vi "BezierGeneratorRev2Trans.vi"(1 "RobotY":dbl, 2 "RobotX":dbl, 3 "DeltaYaw":dbl, 4 "RobotOrientation":dbl=70.0, 5 "DeltaY":dbl=60.0, 6 "DeltaX":dbl=60.0) -> (0 "RobotNeededPathData":T1={"Path"=[], "MaxVel"=80.0, "MaxAccel"=100.0, "Backwards?"=FALSE, "PointSpacing"=6.0, "LookaheadDist"=13.0, "Speed/Curve"=1.8, "SlowDistanceAtEnd"=0.0, "SlowSpeed"=0.0, "MaxDeAccel"=80.0} {"SlowSpeed" format="%#_13g"; "SlowDistanceAtEnd" format="%#_13g"; "Speed/Curve" format="%#_13g"})   [LabVIEW 2018]
uses:
  Dawgma Programming Library/Controls/PurePursuit/RobotNeededPathData.ctl
panel:
  in  "SlowSpeed":dbl
  in  "SlowDistanceAtEnd":dbl
  in  "Speed/Curve":dbl=1.8
  in  "LookaheadDist":dbl=13.0
  in  "PointSpacing":dbl=6.0
  in  "MaxDeaccel":dbl=80.0
  in  "MaxAccel":dbl=100.0
  in  "MaxVel":dbl=80.0
  out "Curve":cluster{"X":dbl, "Y":dbl}[](graph)
  out "waypoints":cluster{dbl[], dbl[]}(graph)
  in  "TrajPointoffset":dbl=12.0
  in  "TargetOffset":dbl=12.0
  in  "Path":cluster{"x":dbl, "y":dbl}[](array[cluster])=[{"x"=0.0, "y"=0.0}, {"x"=0.0, "y"=0.0}, {"x"=0.0, "y"=0.0}, {"x"=0.0, "y"=0.0}]
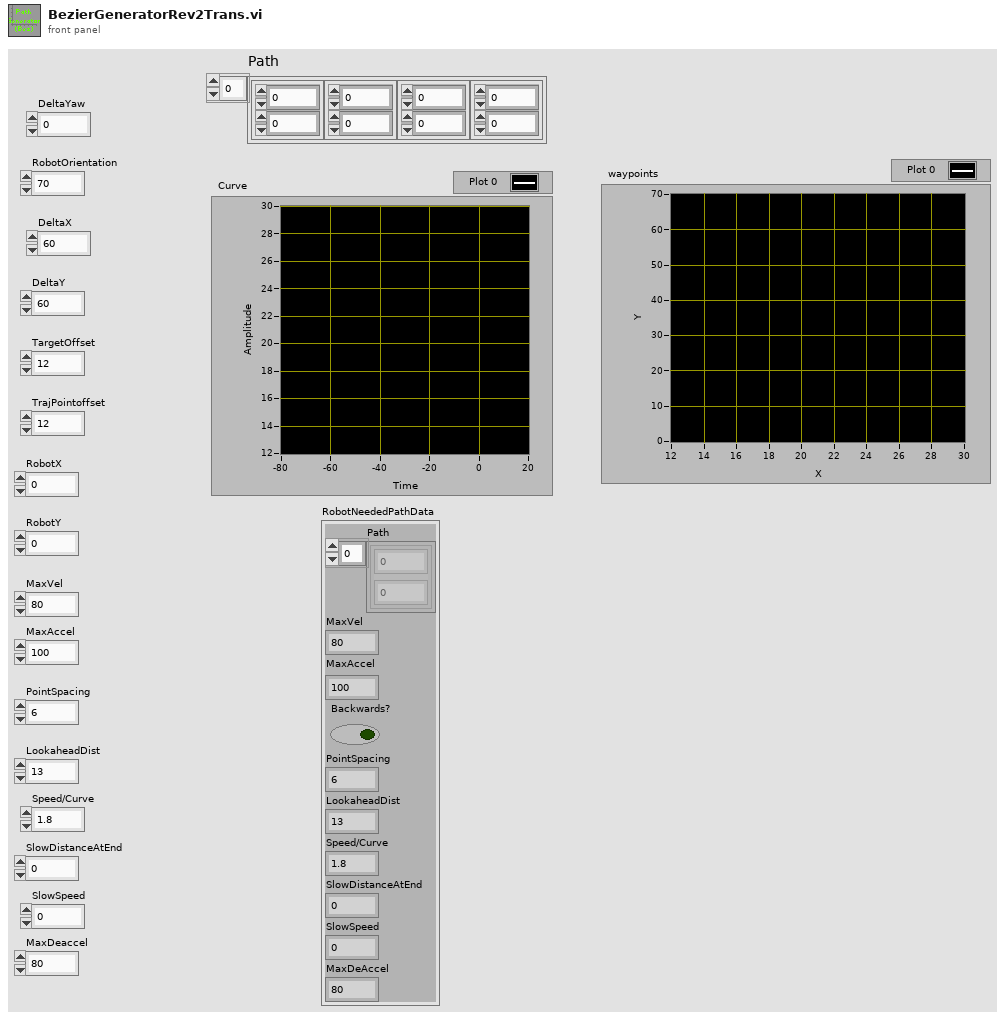
[diagram p1: front panel]
types:
  T1 = typedef "RobotNeededPathData.ctl" = cluster{"Path":cluster{dbl, dbl}[], "MaxVel":dbl, "MaxAccel":dbl, "Backwards?":bool, "PointSpacing":dbl, "LookaheadDist":dbl, "Speed/Curve":dbl, "SlowDistanceAtEnd":dbl, "SlowSpeed":dbl, "MaxDeAccel":dbl}
  T2 = cluster{"DeltaX":dbl, "DeltaY":dbl, "RobotOrientation":dbl, "TrajPointoffset":dbl, "TargetOffset":dbl, "DeltaYaw":dbl, "RobotX":dbl, "RobotY":dbl}
  T3 = cluster{cluster{"xP":dbl, "yP":dbl}[], "MaxVel":dbl, "MaxAccel":dbl, bool, "PointSpacing":dbl, "LookaheadDist":dbl, "Speed/Curve":dbl, "SlowDistanceAtEnd":dbl, "SlowSpeed":dbl, "MaxDeaccel":dbl}
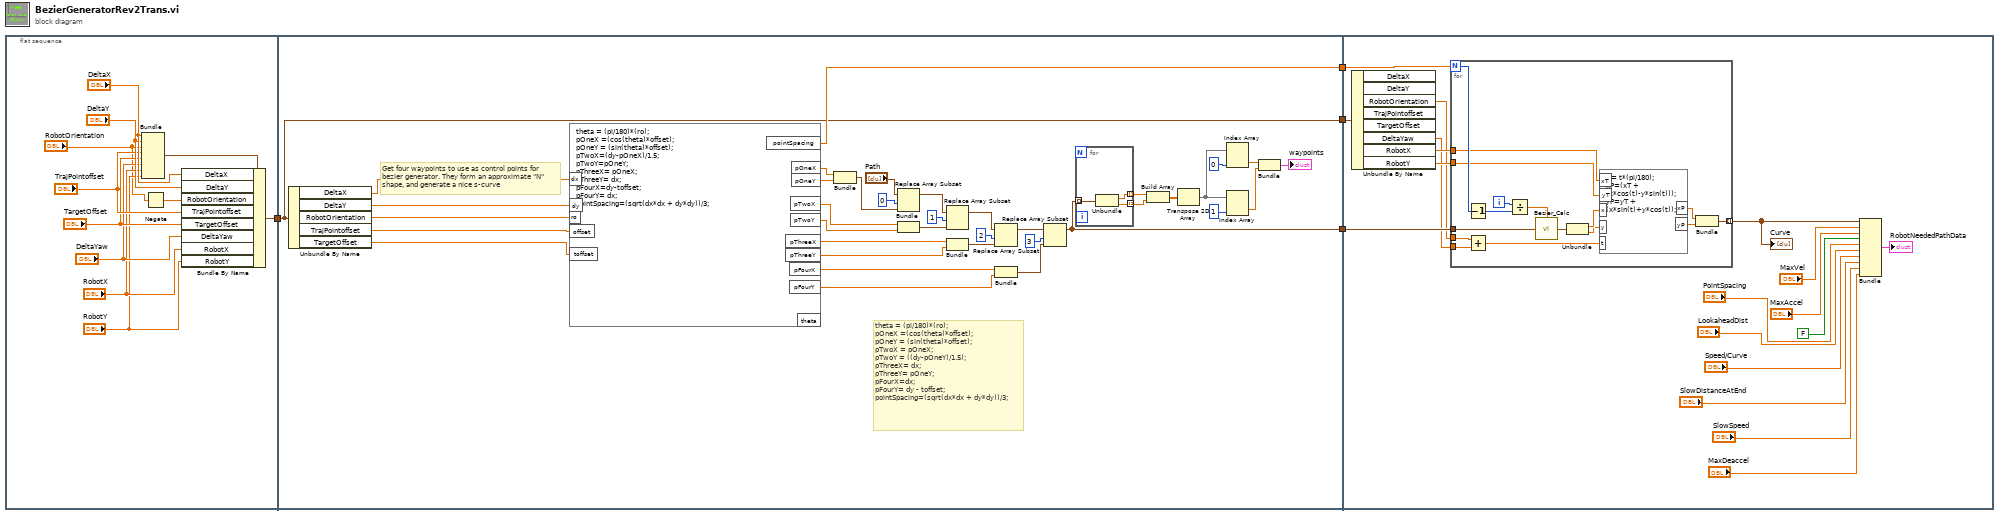
[diagram p0: block diagram]
diagram:
  n1 = flat-sequence {
    tunnel: [w14] -> w2
    tunnel: [w34] -> w4
    tunnel: [w23] -> w3
    tunnel: w2 -> [w16]
    tunnel: [w16] -> w1
    tunnel: w4 -> [w73]
    tunnel: w3 -> [w72]
    tunnel: w1 -> [w61]
    frame #0 {
      n2 = Bundle("DeltaX"="DeltaX", "DeltaY"="DeltaY", "RobotOrientation"="RobotOrientation", "TrajPointoffset"="TrajPointoffset", "TargetOffset"="TargetOffset", "DeltaYaw"="DeltaYaw", "RobotX"="RobotX", "RobotY"="RobotY") -> (w15:T2)  [unwired: 1 in]
      n3 = Negate(x="RobotOrientation") -> (-x=w5:dbl)
      n4 = Bundle By Name(cluster=w15, "DeltaX"="DeltaX", "DeltaY"="DeltaY", "RobotOrientation"=w5, "TrajPointoffset"="TrajPointoffset", "TargetOffset"="TargetOffset", "DeltaYaw"="DeltaYaw", "RobotX"="RobotX", "RobotY"="RobotY") -> (w14:T2)
    }
    frame #1 {
      # "theta = (pi/180)*(ro);\npOneX =(cos(theta)*offset);\npOneY = (sin(theta)*offset);\npTwoX = pOneX;\npTwoY = ((dy-pOneY)/1.5);\npThreeX= dx;\npThreeY= pOneY;\npFourX=dx;\npFourY= dy - toffset;\npointSpacing=(sqrt(dx*dx + dy*dy))/3;"
      # "Get four waypoints to use as control points for bezier generator. They form an approximate \"N\" shape, and generate a nice s-curve"
      n5 = Unbundle By Name(w16) -> ("DeltaX"=w28:dbl, "DeltaY"=w27:dbl, "RobotOrientation"=w24:dbl, "TrajPointoffset"=w25:dbl, "TargetOffset"=w26:dbl)
      n6 = formula code="theta = (pi/180)*(ro);\npOneX =(cos(theta)*offset);\npOneY = (sin(theta)*offset);\npTwoX=(dy-pOneX)/1.5;\npTwoY=pOneY;\npThreeX= pOneX;\npThreeY= dx;\npFourX=dy-toffset;\npFourY= dx;\npointSpacing=(sqrt(dx*dx + dy*dy))/3;"("ro"=w24, "dx"=w28, "dy"=w27, "offset"=w25, "toffset"=w26) -> ("pOneX"=w32:dbl, "pOneY"=w31:dbl, "pTwoX"=w30:dbl, "pTwoY"=w29:dbl, "pointSpacing"=w23:dbl, "pThreeX"=w22:dbl, "pThreeY"=w21:dbl, "pFourX"=w20:dbl, "pFourY"=w19:dbl)  [unwired: 1 out]
      n7 = Bundle("pOneX"=w32, "pOneY"=w31) -> (w43:cluster{"pOneX":dbl, "pOneY":dbl})  [unwired: 1 in]
      n8 = Replace Array Subset(array="Path", new element=w43, index=0) -> (w49:cluster{"x":dbl, "y":dbl}[])
      n9 = Bundle("pTwoX"=w30, "pTwoY"=w29) -> (w44:cluster{"pTwoX":dbl, "pTwoY":dbl})  [unwired: 1 in]
      n10 = Replace Array Subset(array=w49, new element=w44, index=1) -> (w47:cluster{"x":dbl, "y":dbl}[])
      n11 = Bundle("pThreeX"=w22, "pThreeY"=w21) -> (w17:cluster{"pThreeX":dbl, "pThreeY":dbl})  [unwired: 1 in]
      n12 = Replace Array Subset(array=w47, new element=w17, index=2) -> (w45:cluster{"x":dbl, "y":dbl}[])
      n13 = Bundle("pFourX"=w20, "pFourY"=w19) -> (w18:cluster{"pFourX":dbl, "pFourY":dbl})  [unwired: 1 in]
      n14 = Replace Array Subset(array=w45, new element=w18, index=3) -> (w34:cluster{"x":dbl, "y":dbl}[])
      n15 = for {
        tunnel: w34 -> [w55] mode=indexing
        tunnel: [w54] -> w42 mode=indexing
        tunnel: [w53] -> w41 mode=indexing
        n16 = Unbundle(w55) -> ("x"=w54:dbl, "y"=w53:dbl)
      }
      n17 = Build Array(w42, w41) -> (w40:dbl[][])
      n18 = Transpose 2D Array(2D array=w40) -> (transposed array=w37:dbl[][])
      n19 = Index Array(array=w37, index (col)=0 ("disabled index (col)")) -> (element=w35:dbl[])  [unwired: 1 in]
      n20 = Index Array(array=w37, index (col)=1 ("disabled index (col)")) -> (element=w36:dbl[])  [unwired: 1 in]
      n21 = Bundle(w35, w36) -> (→"waypoints":cluster{dbl[], dbl[]})  [unwired: 1 in]
    }
    frame #2 {
      n22 = Unbundle By Name(w61) -> ("RobotOrientation"=w58:dbl, "DeltaYaw"=w57:dbl, "RobotX"=w60:dbl, "RobotY"=w59:dbl)  [unwired: 4 out]
      n23 = for {
        N: w72 -> [w89]
        tunnel: w73 -> [w85]
        tunnel: [w74] -> w56 mode=indexing
        tunnel: w60 -> [w84]
        tunnel: w59 -> [w83]
        tunnel: w58 -> [w79]
        tunnel: w57 -> [w78]
        i -> [w88]
        n24 = Decrement(x=w89) -> (x-1=w87:i32)
        n25 = Add(x=w79, y=w78) -> (x+y=w77:dbl)
        n26 = Divide(x=w88, y=w87) -> (x/y=w86:dbl)
        n27 = call "Bezier_Calc.vi"("points"=w85, "t"=w86) -> ("point out"=w82:cluster{"x":dbl, "y":dbl})
        n28 = Unbundle(w82) -> ("x"=w81:dbl, "y"=w80:dbl)
        n29 = formula code="t = t*(pi/180);\nxP=(xT + (x*cos(t)-y*sin(t)));\nyP=yT + (x*sin(t)+y*cos(t));"("x"=w81, "y"=w80, "t"=w77, "xT"=w84, "yT"=w83) -> ("yP"=w75:dbl, "xP"=w76:dbl)
        n30 = Bundle("xP"=w76, "yP"=w75) -> (w74:cluster{"xP":dbl, "yP":dbl})  [unwired: 1 in]
      }
      "Curve" <- w56
      n31 = Bundle(w56, "MaxVel"="MaxVel", "MaxAccel"="MaxAccel", FALSE, "PointSpacing"="PointSpacing", "LookaheadDist"="LookaheadDist", "Speed/Curve"="Speed/Curve", "SlowDistanceAtEnd"="SlowDistanceAtEnd", "SlowSpeed"="SlowSpeed", "MaxDeaccel"="MaxDeaccel") -> (→"RobotNeededPathData":T3)  [unwired: 1 in]
    }
  }
